vi "DepthSense NewFrame Callback.vi"(4 "User Parameter":T1, 6 "Control Ref":refnum<k24>, 7 "Event Common Data":T2) -> ()   [LabVIEW 2011]
uses:
  C:/Users/Behavior Room/Desktop/Kinect Mouse/DepthSense/FunctionPointerProxy/FunctionPointerProxy/bin/Release/FunctionPointerProxy.dll
  FunctionPointerProxy/FunctionPointerProxy/bin/Release/FunctionPointerProxy.dll
  <vilib>/vision/Image Controls.llb/IMAQ Image.ctl
  <userlib>/libOptrima-2-3/libOptrima-2-3.lvlib
panel:
  in  "queue in":refnum<queue>
  in  "Debug?":bool
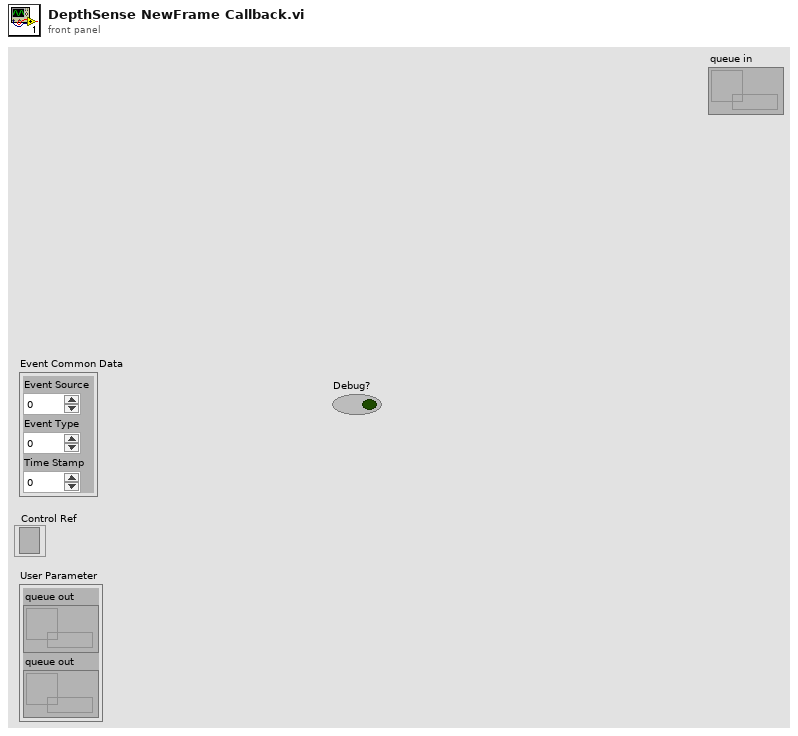
[diagram p1: front panel]
types:
  T1 = cluster{"queue out":refnum<queue>, "queue out":refnum<queue>}
  T2 = cluster{"Event Source":i32, "Event Type":u32, "Time Stamp":u32}
  T3 = typedef "Image Type" = u32
  T4 = typedef "IMAQ Image.ctl" = refnum<image>
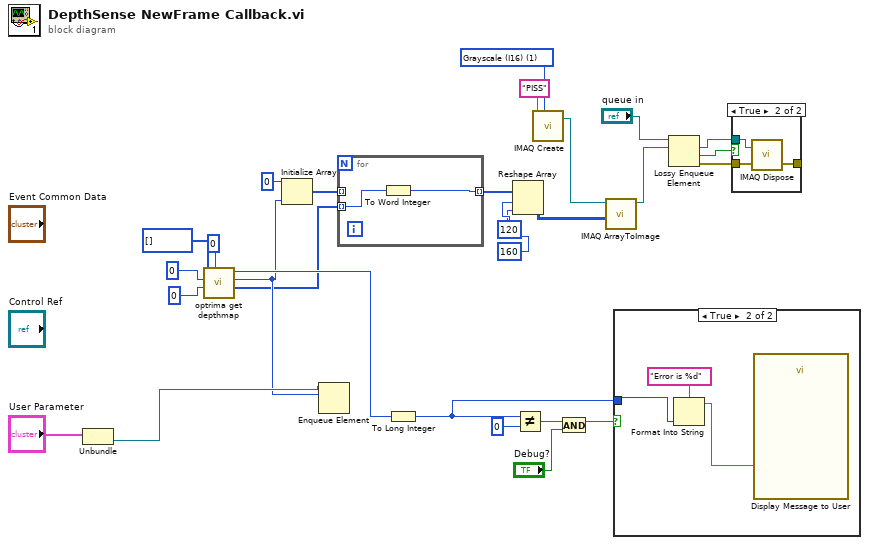
[diagram p0: block diagram]
diagram:
  w16 = T3 1 items=["Grayscale (U8)", "Grayscale (I16)", "Grayscale (SGL)", "Complex (CSG)", "RGB (U32)", "HSL (U32)", "RGB (U64)", "Grayscale (U16)"] ("Image Type")
  n1 = Unbundle("User Parameter") -> ("queue out"=w18:refnum<queue>)  [unwired: 1 out]
  n2 = call <userlib>:"optrima get depthmap.vi"("to_camera_plane"=0, "confidenceTH"=i16 0 ("confidence_threshold"), "length"=u32 0, "p_depthmap in"=u16[] []) -> ("p_depthmap out"=w2:u16[], "length out"=w6:u32, "function return"=w24:u32)  [unwired: 4 in, 1 out]
  n3 = Initialize Array(i16 0 ("element"), w6) -> (w4:i16[])
  n4 = Enqueue Element(queue=w18, element=w6) -> ()  [unwired: 2 in, 3 out]
  n5 = for {
    tunnel: [w29] -> w3 mode=indexing
    tunnel: w4 -> [_] mode=indexing
    tunnel: w2 -> [w30] mode=indexing
    n6 = To Word Integer(number=w30) -> (16bit integer=w29:i16)
  }
  n7 = To Long Integer(number=w24) -> (32bit integer=w22:i32)
  n8 = Reshape Array(w3, 120 ("dimension size"), 160 ("dimension size")) -> (w5:i16[][])
  n9 = Not Equal?(x=w22, y=0) -> (x != y?=w20:bool)
  n10 = call "IMAQ Create"("Image Name"="PISS", "Image Type"=w16) -> ("New Image"=w17:T4)  [unwired: 3 in, 1 out]
  n11 = And(x=w20, y="Debug?") -> (x .and. y?=w21:bool)
  n12 = call "IMAQ ArrayToImage"("Image Pixels (I16)"=w5, "Image"=w17) -> ("Image Out"=w14:T4)  [unwired: 8 in, 1 out]
  n13 = case shown="True" w21 {
    tunnel: w22 -> [_ w31]
    frame False {
    }
    frame True {
      n14 = Format Into String(format string="Error is %d", w31) -> (resulting string=w33:string)  [unwired: 2 in, 1 out]
      n15 = call "Display Message to User"("Message"=w33) -> ()  [unwired: 9 in, 2 out]
    }
  }
  n16 = Lossy Enqueue Element(queue="queue in", element=w14) -> (overflow element=w10:T4, overflow?=w12:bool, error out=w11:errorcluster)  [unwired: 1 in, 1 out]
  n17 = case shown="True" w12 {
    tunnel: w11 -> [w34 w37]
    tunnel: [w34 w36] -> _
    tunnel: w10 -> [_ w35]
    frame False {
    }
    frame True {
      n18 = call "IMAQ Dispose"("Image"=w35, "error in (no error)"=w37) -> ("error out"=w36:errorcluster)  [unwired: 4 in]
    }
  }
